vi "Draw Linear Inverted Pendulum_sim.vi"(1 "Linear Pos and Angle":dbl[](array[numeric])) -> (4 "Unstable?":bool, 5 "Scene.New Object":refnum<vi>)   [LabVIEW 2015]
doc: "This VI draws the Flexible Joint using the \"LabVIEW 3D Picture Control Evaluation Software\".\nThe evaluation software can be downloaded from the following URL: http://digital.ni.com/express.nsf/express?openagent&code=exn4gy"
uses:
  <vilib>/picture/3D Picture Control/NI_3D Picture Control.lvlib
panel:
  out "3D Picture Control":refnum<vi>(3d-picture)
  in  "Reset?":bool
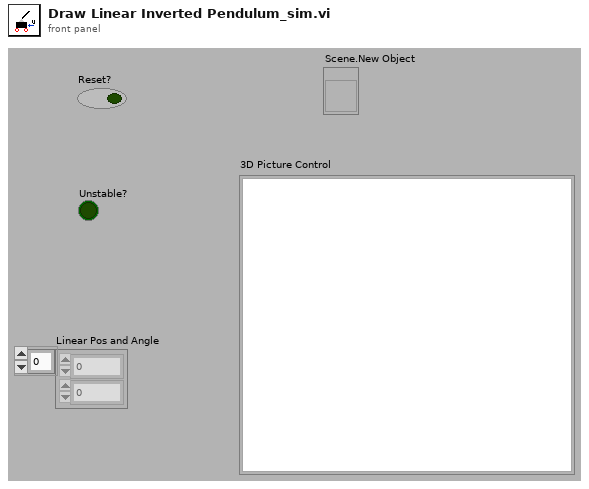
[diagram p1: front panel]
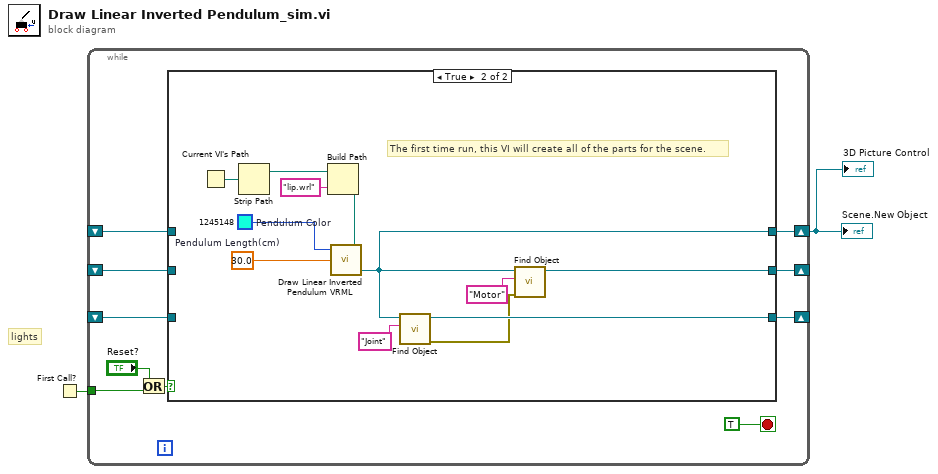
[diagram p0: block diagram]
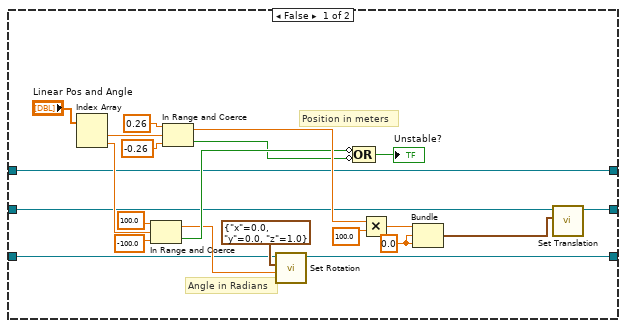
[diagram p2: hidden frame]
diagram:
  # "lights"
  n1 = First Call?() -> (First Call?: T/F=w2:bool)
  n2 = while {
    shift-right: [w4] -> w1
    shift-left: _ -> [w3]
    shift-right: [w11] -> _
    shift-left: _ -> [w10]
    shift-right: [w9] -> _
    shift-left: _ -> [w8]
    tunnel: w2 -> [w5]
    stop <- TRUE stop-if-true
    n3 = Or(x="Reset?", y=w5) -> (x .or. y?=w7:bool)
    n4 = case shown="True" w7 {
      tunnel: [w17 w43] -> w11
      tunnel: w10 -> [w19 _]
      tunnel: [w18 w44] -> w9
      tunnel: w8 -> [w20 _]
      tunnel: [w16 w37] -> w4
      tunnel: w3 -> [w16 _]
      frame False {
        w14 = 0.0
        # "Position in meters"
        # "Angle in Radians"
        n5 = Index Array(array="Linear Pos and Angle") -> (element #1=w28:dbl, element #2=w33:dbl)  [unwired: 2 in]
        n6 = In Range and Coerce(upper limit=100.0, x=w33, lower limit=-100.0) -> (coerced(x)=w22:dbl, In Range?=w25:bool)
        n7 = In Range and Coerce(upper limit=0.26, x=w28, lower limit=-0.26) -> (coerced(x)=w26:dbl, In Range?=w24:bool)
        n8 = call <vilib>:"Set Rotation.vi"("Angle"=w22, "Axis"=cluster{"x":dbl, "y":dbl, "z":dbl} {"x"=0.0, "y"=0.0, "z"=1.0}, "Scene Object"=w20) -> ("Rotated Scene Object"=w18:refnum<vi>)  [unwired: 1 in, 7 out]
        n9 = Compound Arithmetic op=OR(invert w25, invert w24) -> (→"Unstable?":bool)
        n10 = Multiply(x=w26, y=100.0) -> (x*y=w15:dbl)
        n11 = Bundle(w15, w14, w14) -> (w13:cluster{dbl, dbl, dbl})  [unwired: 1 out]
        n12 = call <vilib>:"Set Translation.vi"("Translation"=w13, "Scene Object"=w19) -> ("Translated Object"=w17:refnum<vi>)  [unwired: 1 in, 8 out]
      }
      frame True {
        w39 = u32 1245148  # Pendulum Color
        w38 = 30.0  # Pendulum Length(cm)
        # "The first time run, this VI will create all of the parts for the scene."
        n13 = Current VI's Path() -> (path=w42:path)
        n14 = Strip Path(path=w42) -> (stripped path=w41:path)  [unwired: 1 out]
        n15 = Build Path(base path=w41, name or relative path="lip.wrl") -> (appended path=w36:path)
        n16 = call "Draw Linear Inverted Pendulum VRML.vi"("Path to WRL file"=w36, "Height"=w38, "Pendulum Color"=w39) -> ("Scene.New Object"=w37:refnum<vi>)  [unwired: 2 out]
        n17 = call <vilib>:"Find Object.vi"("Object Name"="Joint" ("Name"), "Scene Refnum"=w37) -> ("error out"=w35:errorcluster, "Object Refnum"=w44:refnum<vi>)  [unwired: 1 in, 7 out]
        n18 = call <vilib>:"Find Object.vi"("error in (no error)"=w35, "Object Name"="Motor" ("Name"), "Scene Refnum"=w37) -> ("Object Refnum"=w43:refnum<vi>)  [unwired: 8 out]
      }
    }
  }
  "Scene.New Object" <- w1
  "3D Picture Control" <- w1
